vi "_FPGA_Digit_in_ones_U4.vi"(10 "LastFourBits":bool[](array[boolean])) -> (2 "DigitInOnes_U6":fxp<+/-,5,5>)   [LabVIEW 2018]
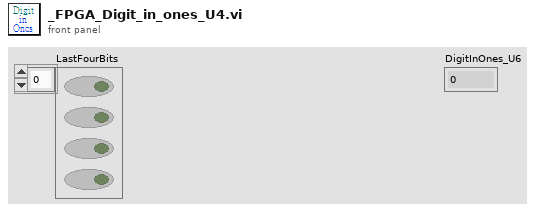
[diagram p1: front panel]
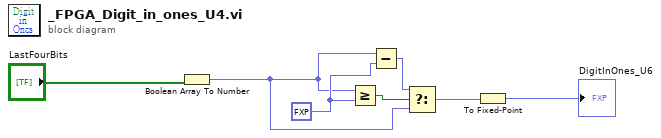
[diagram p0: block diagram]
diagram:
  w5 = fxp<+,4,4> 10.0 ("y")
  n1 = Boolean Array To Number(Boolean array="LastFourBits") -> (number=w3:fxp<+,4,4>)
  n2 = Greater Or Equal?(x=w3, y=w5) -> (x >= y?=w6:bool)
  n3 = Subtract(x=w3, y=w5) -> (x-y=w4:fxp<+/-,5,5>)
  n4 = Select(t=w4, s=w6, f=w3) -> (s? t:f=w2:fxp<+/-,5,5>)
  n5 = To Fixed-Point(number=w2) -> (fixed-point=→"DigitInOnes_U6":fxp<+/-,5,5>)  [unwired: 1 in]
